vi "GTCP331-200ER - 1.C.(3)(4).vi"(8 "error in (no error)":errorcluster, 11 "RT - Analysis Data in in in":T1={"Accel Sensistivity"=[0.0, 0.0, 0.0], "Cutoff Frequncies"=[{"LP Passband"=0.0, "HP Stopband"=0.0, "LP Stopband"=0.0, "HP Passband"=0.0}, {"LP Passband"=0.0, "HP Stopband"=0.0, "LP Stopband"=0.0, "HP Passband"=0.0}, {"LP Passband"=0.0, "HP Stopband"=0.0, "LP Stopband"=0.0, "HP Passband"=0.0}], "APU Setup File"={"Sensor Info"=[], "Calibration Info"=[], "CMM Table 106"=[], "CMM Table 106B "=[], "Accel Config"=[], "Report Sheet 1"=[], "Report Sheet 2"=[], "Report Sheet 3"=[]}, "RepairLevel"=""} {"Cutoff Frequncies"."HP Passband" min=1.0 step=1.0 format="%#.4f"; "Cutoff Frequncies"."LP Stopband" min=1.0 step=1.0 format="%#.4f"; "Cutoff Frequncies"."HP Stopband" min=1.0 step=1.0 format="%#.4f"; "Cutoff Frequncies"."LP Passband" min=1.0 step=1.0 format="%#.4f"}) -> (0 "error out":errorcluster, 2 "Interactive Mode Vals":dbl[](array[numeric]), 3 "RT - Analysis Data in out":T1 {"Cutoff Frequncies"."HP Passband" min=1.0 step=1.0 format="%#.4f"; "Cutoff Frequncies"."LP Stopband" min=1.0 step=1.0 format="%#.4f"; "Cutoff Frequncies"."HP Stopband" min=1.0 step=1.0 format="%#.4f"; "Cutoff Frequncies"."LP Passband" min=1.0 step=1.0 format="%#.4f"})   [LabVIEW 2018, in "RT - Analysis.lvlib"]
doc: "This subtest perfmors engine run-in procedures."
uses:
  RT - Analysis.lvlib
  Public Controls/Alert Data.ctl
  Private Controls/Watchdog Settings.ctl
  Private Controls/Interactive Data.ctl
  <vilib>/Analysis/NI_AALBase.lvlib
  <vilib>/Analysis/baseanly.llb/Mean (DBL).vi
  Private Controls/RT-Analysis Data.ctl
  Modules/Testing UI 3/Private Controls/Cutoff Frequency.ctl
  Modules/Testing UI 3/Testing UI 3.lvlib
  Top Level/Shared Controls/APU Setup File.ctl
panel:
  # "Highpass Cutoff Frequency"
  # "Lowpass Cutoff Frequency"
  # "Highpass Cutoff Frequency"
  # "Lowpass Cutoff Frequency"
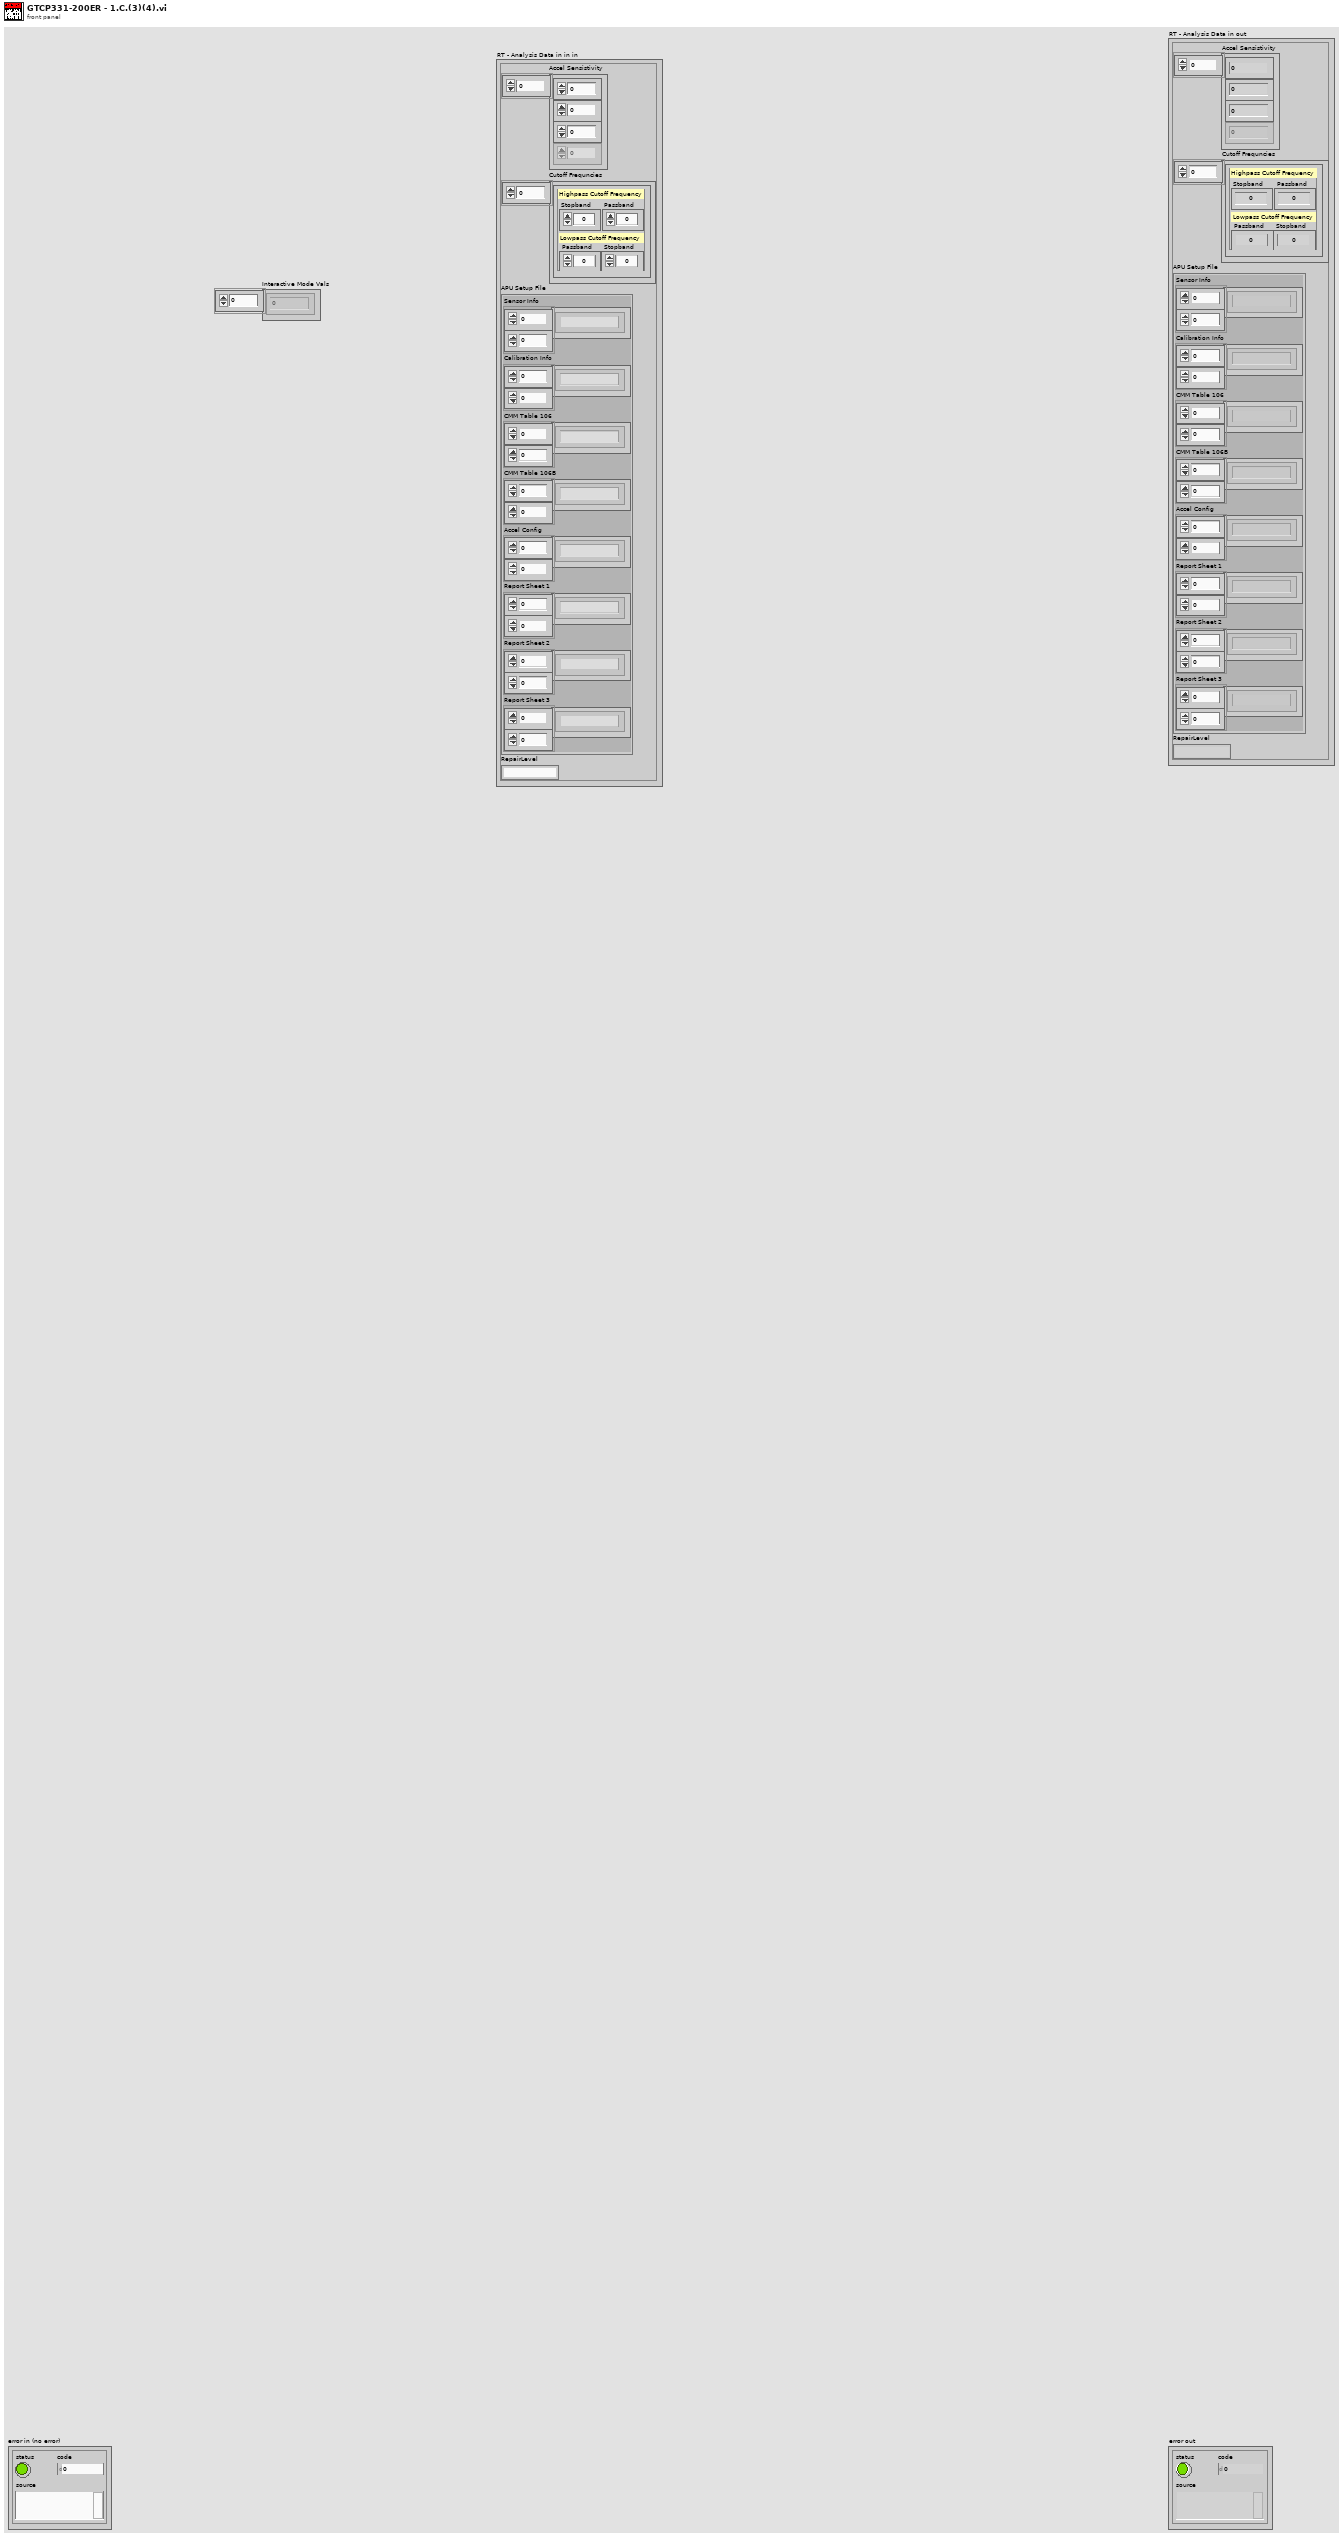
[diagram p1: front panel]
types:
  T1 = typedef "RT - Analysis.lvlib/RT-Analysis Data.ctl" = cluster{"Accel Sensistivity":dbl[], "Cutoff Frequncies":T2[], "APU Setup File":T3, "RepairLevel":string}
  T2 = typedef "Testing UI 3.lvlib/Cutoff Frequency.ctl" = cluster{"LP Passband":dbl, "HP Stopband":dbl, "LP Stopband":dbl, "HP Passband":dbl}
  T3 = typedef "APU Setup File.ctl" = cluster{"Sensor Info":string[][], "Calibration Info":string[][], "CMM Table 106":string[][], "CMM Table 106B ":string[][], "Accel Config":string[][], "Report Sheet 1":string[][], "Report Sheet 2":string[][], "Report Sheet 3":string[][]}
  T4 = typedef "RT - Analysis.lvlib/Alert Data.ctl" = cluster{"Tag":string, "Value":dbl, "Alerts":bool[], "Thresh Val":dbl, "Thresh Len":dbl, "Thresh Type":enum16{"Neither", "Max", "Min"}}
  T5 = typedef "RT - Analysis.lvlib/Watchdog Settings.ctl" = cluster{"Watchdog Action":enum16{"Disabled", "Timer - Change Sample Rate", "RPM Thresh - Insert Other", "RPM Thresh - Check POPD", "RPM Thresh - StartStop Logging"}, "Timer Start":timestamp, "[Watchdog Bools]":bool[], "[Watchdog DBLs]":dbl[], "Watchdog Variant":variant}
  T6 = typedef "RT - Analysis.lvlib/Interactive Data.ctl" = cluster{"Confirm Pressed":bool, "Stored Vals":dbl[]}
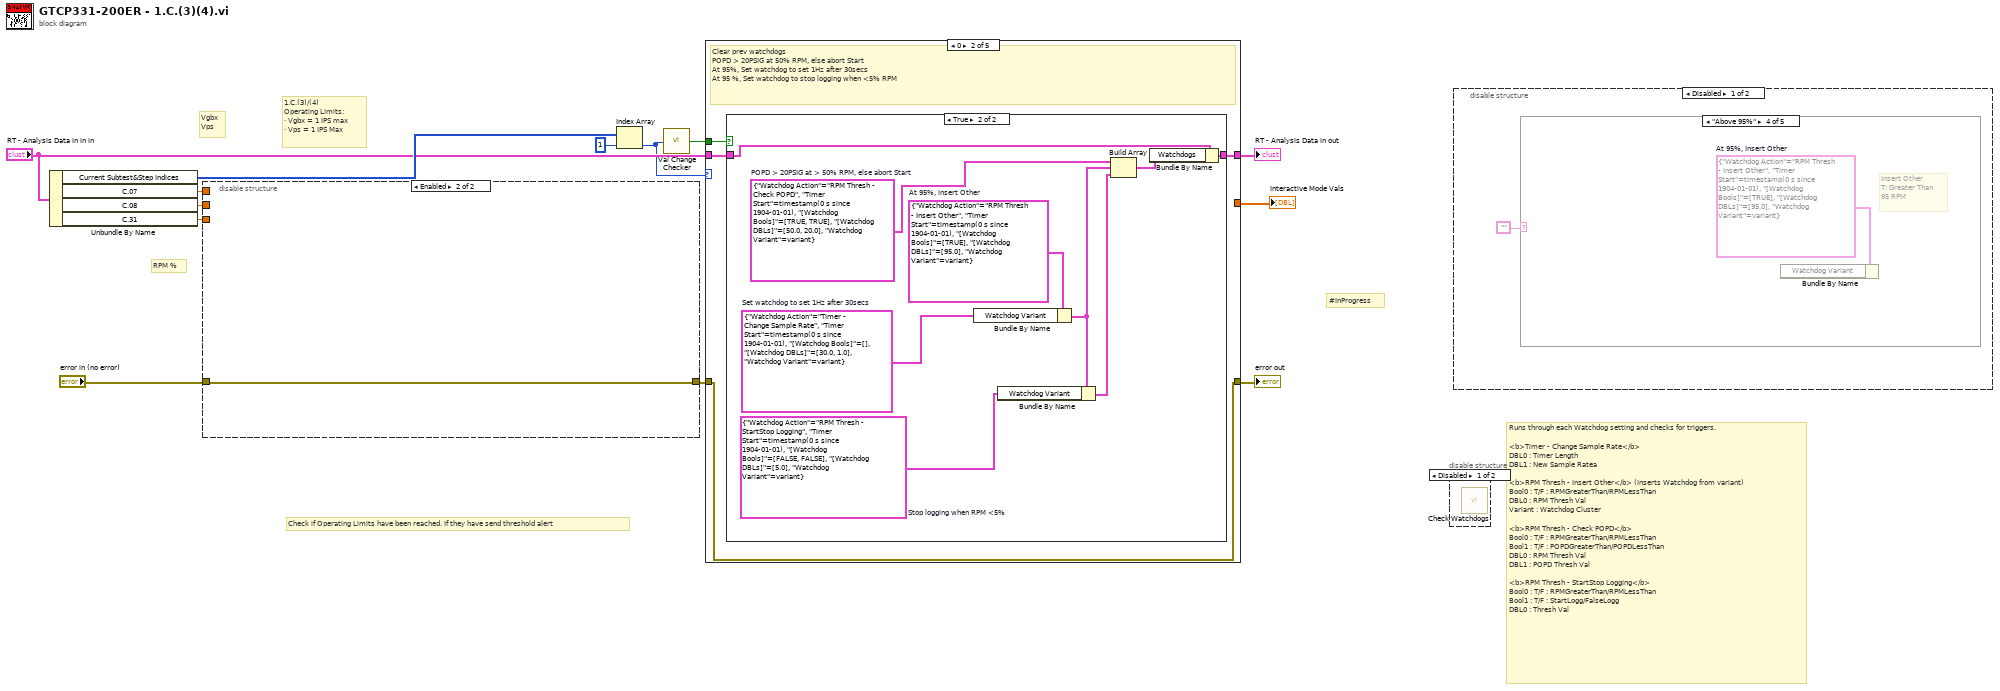
[diagram p0: block diagram]
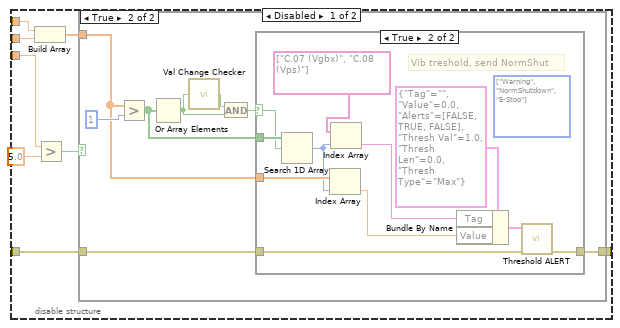
[diagram p2: hidden frame]
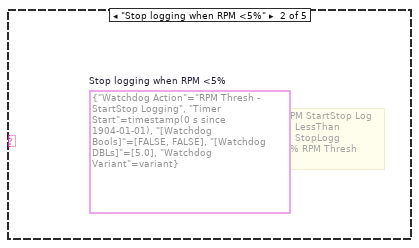
[diagram p6: hidden frame]
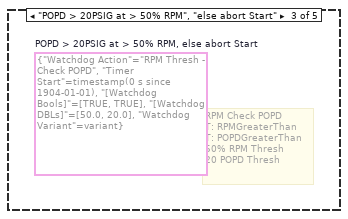
[diagram p7: hidden frame]
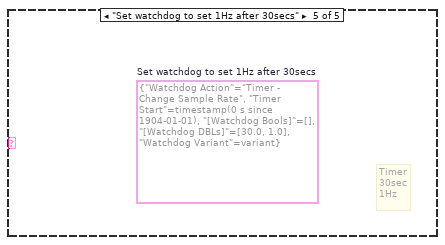
[diagram p8: hidden frame]
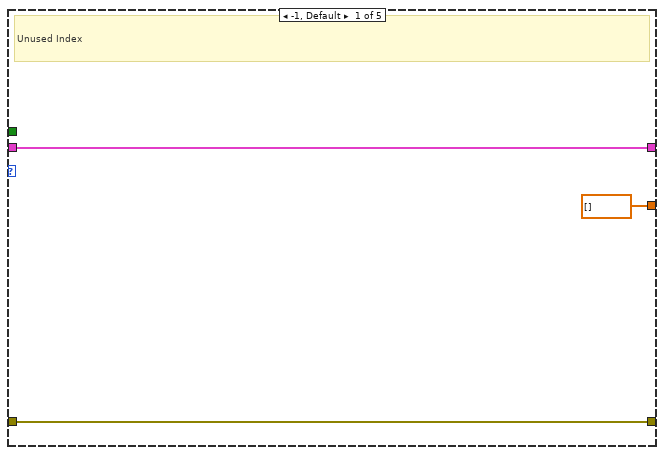
[diagram p11: hidden frame]
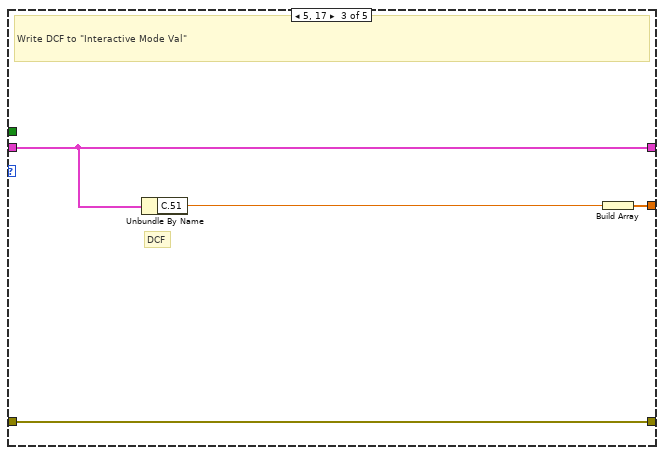
[diagram p13: hidden frame]
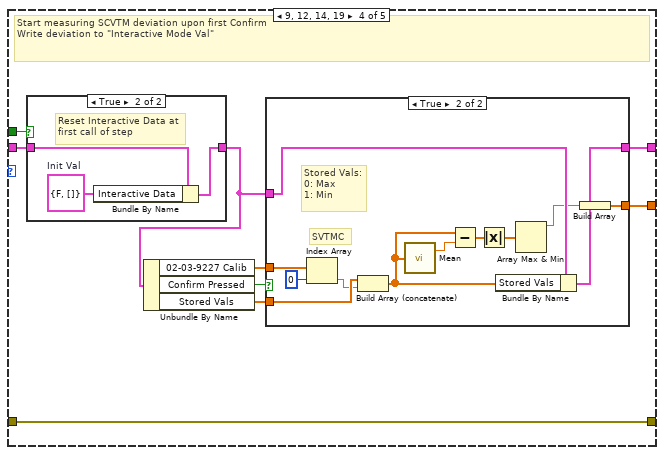
[diagram p14: hidden frame]
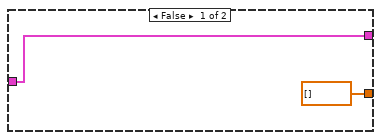
[diagram p15: hidden frame]
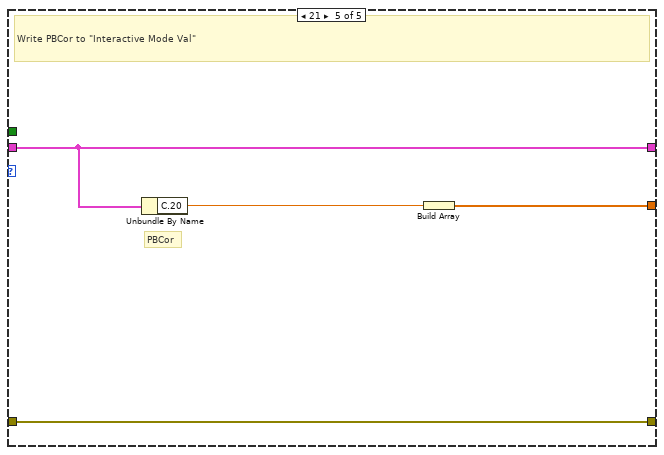
[diagram p17: hidden frame]
diagram:
  # "RPM %"
  # "#InProgress"
  # "Runs through each Watchdog setting and checks for triggers.\n\n<b>Timer - Change Sample Rate</b>\nDBL0 : Timer Length\nDBL1 : New Sample Ratea\n\n<b>RPM Thresh - Insert Other</b> (Inserts Watchdog from variant)\nBool0 : T/F : RPMGreaterThan/RPMLessThan\nDBL0 : RPM Thresh Val\nVariant : Watchdog Cluster\n\n<b>RPM Thresh - Check POPD</b>\nBool0 : T/F : RPMGreaterThan/RPMLessThan\nBool1 : T/F : POPDGreaterThan/POPDLessThan\nDBL0 : RPM Thresh Val\nDBL1 : POPD Thresh Val\n\n<b>RPM Thresh - StartStop Logging</b>\nBool0 : T/F : RPMGreaterThan/RPMLessThan\nBool1 : T/F : StartLogg/FalseLogg\nDBL0 : Thresh Val"
  # "Check if Operating Limits have been reached. If they have send threshold alert"
  # "Vgbx\nVps"
  # "1.C.(3)/(4)\nOperating Limits:\n· Vgbx = 1 IPS max\n· Vps = 1 IPS Max"
  n1 = Unbundle By Name("RT - Analysis Data in in in") -> ("Current Subtest&Step Indices"=w13:i32[], "C.07"=w9:dbl, "C.08"=w8:dbl, "C.31"=w2:dbl)
  n2 = disable-structure shown="Enabled" {
    disable-tunnel: w9 -> [w21 _]
    disable-tunnel: w8 -> [w20 _]
    disable-tunnel: [w19 w43] -> w7
    disable-tunnel: "error in (no error)" -> [w17 w43]
    disable-tunnel: w2 -> [w15 _]
    frame Disabled {
      n3 = Build Array(w21, w20) -> (w18:dbl[])
      n4 = Greater?(x=w15, y=5.0) -> (0:w16:bool)
      n5 = case shown="True" w16 {
        tunnel: [w22 w29] -> w19
        tunnel: w18 -> [_ w27]
        tunnel: w17 -> [w22 w23]
        frame False {
        }
        frame True {
          n6 = Greater?(x=w27, y=1 ("C.08")) -> (0:w28:bool[])
          n7 = Or Array Elements(Boolean array=w28) -> (logical OR=w25:bool)
          n8 = call "Val Change Checker.vi"("Current Value in"=w25) -> ("Value Change?"=w26:bool)
          n9 = And(x=w26, y=w25) -> (x .and. y?=w24:bool)
          n10 = case shown="True" w24 {
            selector: w24 -> [_ w41]
            tunnel: w23 -> [w31 w37]
            tunnel: [w31 w36] -> w29
            tunnel: w28 -> [_ w42]
            tunnel: w27 -> [_ w40]
            frame False {
            }
            frame True {
              (unwired) enum32{"Warning", "NormShutdown", "E-Stop"}[] [enum."Warning", enum."NormShutdown", enum."E-Stop"] items=["Warning", "NormShutdown", "E-Stop"]
              # "Vib treshold, send NormShut"
              n11 = Search 1D Array(1D array=w42, element=w41) -> (index of element=w39:i32)  [unwired: 1 in]
              n12 = Index Array(array=w40, index=w39) -> (element=w32:dbl)
              n13 = Index Array(array=string[] ["C.07 (Vgbx)", "C.08 (Vps)"], index=w39) -> (element=w33:string)
              n14 = Bundle By Name(cluster=T4 {"Tag"="", "Value"=0.0, "Alerts"=[FALSE, TRUE, FALSE], "Thresh Val"=1.0, "Thresh Len"=0.0, "Thresh Type"=enum."Max"} ("Alert Data"), "Tag"=w33, "Value"=w32) -> (w35:T4)
              n15 = call "Threshold ALERT.vi"("error in (no error)"=w37, "Alert Data"=w35) -> ("error out"=w36:errorcluster)  [unwired: 9 in]
            }
          }
        }
      }
    }
    frame Enabled {
    }
  }
  n16 = Index Array(array=w13, index=1) -> (element=w4:i32)
  n17 = call "Val Change Checker.vi"("Current Value in"=w4) -> ("Value Change?"=w3:bool)
  n18 = case shown="0" w4 {
    tunnel: [w46 w50 w64 w73 w95] -> w11
    tunnel: w7 -> [w46 w50 w64 w73 w95]
    tunnel: [w45 w49 w63 w66 w94] -> w10
    tunnel: "RT - Analysis Data in in in" -> [w45 w48 w63 w70 w94]
    tunnel: [dbl[] [] ("Interactive Mode Vals") _ w61 w72 w92] -> w1
    tunnel: w3 -> [_ w47 _ w71 _]
    frame -1, Default {
      # "Unused Index"
    }
    frame 0 {
      # "Clear prev watchdogs\nPOPD > 20PSIG at 50% RPM, else abort Start\nAt 95%, Set watchdog to set 1Hz after 30secs\nAt 95 %, Set watchdog to stop logging when <5% RPM"
      n19 = case shown="True" w47 {
        tunnel: [w51 w60] -> w49
        tunnel: w48 -> [w51 w59]
        frame False {
        }
        frame True {
          w52 = T5 {"Watchdog Action"=enum."RPM Thresh - StartStop Logging", "Timer Start"=timestamp(0 s since 1904-01-01), "[Watchdog Bools]"=[FALSE, FALSE], "[Watchdog DBLs]"=[5.0], "Watchdog Variant"=variant}  # Stop logging when RPM <5%
          w57 = T5 {"Watchdog Action"=enum."Timer - Change Sample Rate", "Timer Start"=timestamp(0 s since 1904-01-01), "[Watchdog Bools]"=[], "[Watchdog DBLs]"=[30.0, 1.0], "Watchdog Variant"=variant}  # Set watchdog to set 1Hz after 30secs
          w56 = T5 {"Watchdog Action"=enum."RPM Thresh - Insert Other", "Timer Start"=timestamp(0 s since 1904-01-01), "[Watchdog Bools]"=[TRUE], "[Watchdog DBLs]"=[95.0], "Watchdog Variant"=variant}  # At 95%, Insert Other
          w55 = T5 {"Watchdog Action"=enum."RPM Thresh - Check POPD", "Timer Start"=timestamp(0 s since 1904-01-01), "[Watchdog Bools]"=[TRUE, TRUE], "[Watchdog DBLs]"=[50.0, 20.0], "Watchdog Variant"=variant}  # POPD > 20PSIG at > 50% RPM, else abort Start
          n20 = Bundle By Name(cluster=w56, "Watchdog Variant"=w57) -> (w54:T5)
          n21 = Bundle By Name(cluster=w54, "Watchdog Variant"=w52) -> (w53:T5)
          n22 = Build Array(w55, w54, w53) -> (w58:T5[])
          n23 = Bundle By Name(cluster=w59, "Watchdogs"=w58) -> (w60:T1)
        }
      }
    }
    frame 5, 17 {
      # "DCF"
      # "Write DCF to \"Interactive Mode Val\""
      n24 = Unbundle By Name(w63) -> ("C.51"=w62:dbl)
      n25 = Build Array(w62) -> (w61:dbl[])
    }
    frame 9, 12, 14, 19 {
      # "Start measuring SCVTM deviation upon first Confirm\nWrite deviation to \"Interactive Mode Val\""
      n26 = case shown="True" w71 {
        tunnel: w70 -> [w88 w91]
        tunnel: [w88 w90] -> w69
        frame False {
        }
        frame True {
          w89 = T6 {"Confirm Pressed"=FALSE, "Stored Vals"=[]}  # Init Val
          # "Reset Interactive Data at\nfirst call of step"
          n27 = Bundle By Name(cluster=w91, "Interactive Data"=w89) -> (w90:T1)
        }
      }
      n28 = Unbundle By Name(w69) -> ("02-03-9227 Calib"=w65:dbl[], "Confirm Pressed"=w68:bool, "Stored Vals"=w67:dbl[])
      n29 = case shown="True" w68 {
        tunnel: [dbl[] [] ("Interactive Mode Vals") w76] -> w72
        tunnel: w69 -> [w75 w87]
        tunnel: w67 -> [_ w83]
        tunnel: [w75 w86] -> w66
        tunnel: w65 -> [_ w85]
        frame False {
        }
        frame True {
          # "Stored Vals:\n0: Max\n1: Min"
          # "SVTMC"
          n30 = Index Array(array=w85, index=0) -> (element=w82:dbl)
          n31 = Build Array (concatenate)(w83, w82) -> (w80:dbl[])
          n32 = call-poly <vilib>:"Mean.vi"("X"=w80) -> ("mean"=w81:dbl)  [unwired: 1 out]
          n33 = Subtract(x=w80, y=w81) -> (x-y=w79:dbl[])
          n34 = Absolute Value(x=w79) -> (abs(x)=w78:dbl[])
          n35 = Bundle By Name(cluster=w87, "Stored Vals"=w80) -> (w86:T1)
          n36 = Array Max & Min(array=w78) -> (max value=w77:dbl)  [unwired: 3 out]
          n37 = Build Array(w77) -> (w76:dbl[])
        }
      }
    }
    frame 21 {
      # "PBCor"
      # "Write PBCor to \"Interactive Mode Val\""
      n38 = Unbundle By Name(w94) -> ("C.20"=w93:dbl)
      n39 = Build Array(w93) -> (w92:dbl[])
    }
  }
  "RT - Analysis Data in out" <- w10
  "error out" <- w11
  "Interactive Mode Vals" <- w1
  n40 = disable-structure shown="Disabled" {
    frame Disabled {
      n41 = call "Check Watchdogs.vi"() -> ()  [unwired: 10 in, 2 out]
    }
    frame Enabled {
    }
  }
  n42 = disable-structure shown="Disabled" {
    frame Disabled {
      n43 = case shown="\"Above 95%\"" "" {
        frame Default {
        }
        frame "Stop logging when RPM <5%" {
          (unwired) T5 {"Watchdog Action"=enum."RPM Thresh - StartStop Logging", "Timer Start"=timestamp(0 s since 1904-01-01), "[Watchdog Bools]"=[FALSE, FALSE], "[Watchdog DBLs]"=[5.0], "Watchdog Variant"=variant}  # Stop logging when RPM <5%
          # "RPM StartStop Log\nF: LessThan\nF: StopLogg\n5% RPM Thresh"
        }
        frame "POPD > 20PSIG at > 50% RPM", "else abort Start" {
          (unwired) T5 {"Watchdog Action"=enum."RPM Thresh - Check POPD", "Timer Start"=timestamp(0 s since 1904-01-01), "[Watchdog Bools]"=[TRUE, TRUE], "[Watchdog DBLs]"=[50.0, 20.0], "Watchdog Variant"=variant}  # POPD > 20PSIG at > 50% RPM, else abort Start
          # "RPM Check POPD\nT: RPMGreaterThan\nT: POPDGreaterThan\n50% RPM Thresh\n20 POPD Thresh"
        }
        frame "Above 95%" {
          w97 = T5 {"Watchdog Action"=enum."RPM Thresh - Insert Other", "Timer Start"=timestamp(0 s since 1904-01-01), "[Watchdog Bools]"=[TRUE], "[Watchdog DBLs]"=[95.0], "Watchdog Variant"=variant}  # At 95%, Insert Other
          # "Insert Other\nT: Greater Than\n95 RPM"
          n44 = Bundle By Name(cluster=w97) -> ()  [unwired: 1 in, 1 out]
        }
        frame "Set watchdog to set 1Hz after 30secs" {
          (unwired) T5 {"Watchdog Action"=enum."Timer - Change Sample Rate", "Timer Start"=timestamp(0 s since 1904-01-01), "[Watchdog Bools]"=[], "[Watchdog DBLs]"=[30.0, 1.0], "Watchdog Variant"=variant}  # Set watchdog to set 1Hz after 30secs
          # "Timer\n30sec\n1Hz"
        }
      }
    }
    frame Enabled {
    }
  }
